vi "Read.vi"(8 "error in (no error)":errorcluster, 9 "Starting independent variables":dbl[](array[numeric]), 10 "Current independent variables":dbl[](array[numeric]), 11 "Photon Counter with LCD Reader in":refnum<class "Photon Counter with LCD Reader.lvclass">) -> (0 "error out":errorcluster, 2 "Data Channels":T1, 3 "Photon Counter with LCD Reader out":refnum<class "Photon Counter with LCD Reader.lvclass">)   [LabVIEW 2017, in "Photon Counter with LCD Reader.lvclass"]
doc: "Prepare for read, wait the time delay, and take data from up to 4 channels."
uses:
  Photon Counter with LCD Reader.lvclass
  Instruments/Utility Classes/Readable/Data Channels.ctl
  Instruments/Utility Classes/Readable/Data Channel.ctl
  Instruments/Utility Classes/Readable/Data Point.ctl
  Instruments/Utility Classes/Readable/Time.ctl
  Instruments/Utility Classes/Readable/X.ctl
  Photon Counter with LCD Reader.lvclass/Photon Counter with LCD Reader.ctl
  Reader/Reader.lvclass
  Instruments/LCD/LCD Retarder.lvclass
  Instruments/Utility Classes/Readable/Readable.lvclass
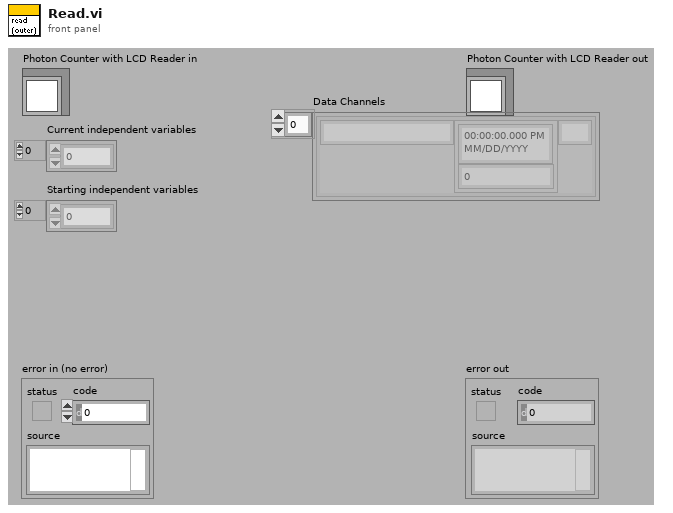
[diagram p1: front panel]
types:
  T1 = typedef "Readable.lvclass/Data Channels.ctl" = T2[]
  T2 = typedef "Readable.lvclass/Data Channel.ctl" = cluster{"Name":string, "Data Point":T3, "Unit":string}
  T3 = typedef "Readable.lvclass/Data Point.ctl" = cluster{"t":T4, "x":T5}
  T4 = typedef "Readable.lvclass/Time.ctl" = timestamp
  T5 = typedef "Readable.lvclass/X.ctl" = dbl
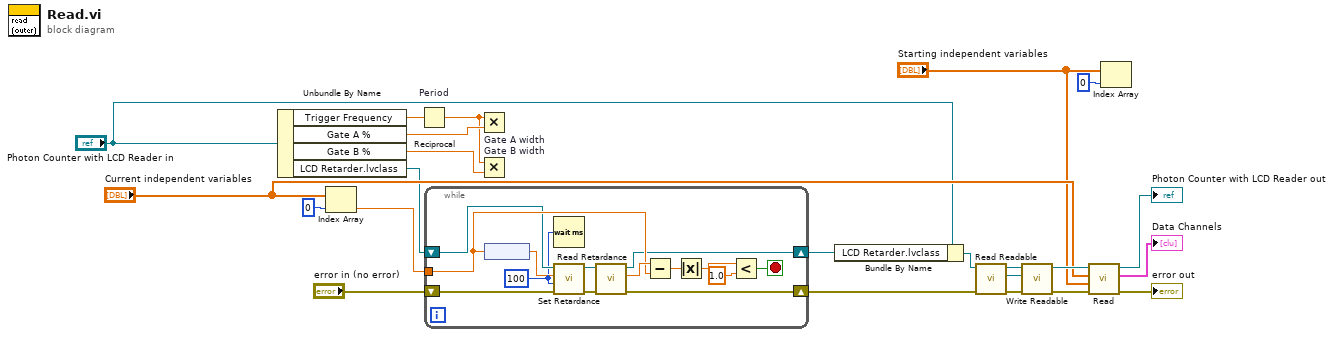
[diagram p0: block diagram]
diagram:
  n1 = Unbundle By Name("Photon Counter with LCD Reader in") -> ("Trigger Frequency"=w19:dbl[unit], "Gate A %"=w18:dbl, "Gate B %"=w17:dbl, "LCD Retarder.lvclass"=w7:refnum<class "LCD Retarder.lvclass">)
  n2 = Index Array(array="Current independent variables", index=0) -> (element=w4:dbl)
  n3 = Reciprocal "Period"(x=w19) -> (1/x=w16:dbl[unit])
  n4 = while {
    tunnel: w4 -> [w32]
    shift-right: [w29] -> w5
    shift-left: "error in (no error)" -> [w28]
    shift-right: [w30] -> w2
    shift-left: w7 -> [w26]
    stop <- w33 stop-if-true
    w24 = u32 100 ("milliseconds to wait")
    n5 = node(w32) -> (w31:dbl[unit])
    n6 = Wait (ms)(milliseconds to wait=w24) -> ()  [unwired: 1 out]
    n7 = call "Set Retardance.vi"("errorIN"=w28, "milliseconds to wait (0)"=w24, "Retardance"=w31, "LCD in"=w26) -> ("errorOUT"=w27:errorcluster, "LCD out"=w25:refnum<class "LCD Retarder.lvclass">)  [unwired: 5 in, 1 out]
    n8 = call "Read Retardance.vi"("errorIN"=w27, "LCD in"=w25) -> ("errorOUT"=w29:errorcluster, "Retardance out"=w37:dbl, "LCD out"=w30:refnum<class "LCD Retarder.lvclass">)  [unwired: 7 in]
    n9 = Subtract(x=w37, y=w32) -> (x-y=w36:dbl)
    n10 = Absolute Value(x=w36) -> (abs(x)=w35:dbl)
    n11 = Less?(x=w35, y=1.0) -> (x < y?=w33:bool)
  }
  n12 = Multiply "Gate A width"(x=w16, y=w18) -> ()  [unwired: 1 out]
  n13 = Multiply "Gate B width"(x=w16, y=w17) -> ()  [unwired: 1 out]
  n14 = Bundle By Name(cluster="Photon Counter with LCD Reader in", "LCD Retarder.lvclass"=w2) -> (w1:refnum<class "Photon Counter with LCD Reader.lvclass">)
  n15 = call-dynamic "Read Readable.vi"("error in (no error)"=w5, "Reader.lvclass in"=w1) -> ("error out"=w13:errorcluster, "Readable.lvclass"=w14:refnum<class "Readable.lvclass">, "Reader.lvclass out"=w15:refnum<class "Photon Counter with LCD Reader.lvclass">)  [unwired: 7 out]
  n16 = call-dynamic "Write Readable.vi"("error in (no error)"=w13, "Readable.lvclass"=w14, "Reader.lvclass in"=w15) -> ("error out"=w9:errorcluster, "Reader.lvclass out"=w12:refnum<class "Photon Counter with LCD Reader.lvclass">)  [unwired: 7 out]
  n17 = call-parent "Read.vi"("error in (no error)"=w9, "Starting independent variables"="Starting independent variables", "Current independent variables"="Current independent variables", "Reader in"=w12) -> ("error out"=→"error out":errorcluster, "Data Channels"=→"Data Channels":T1, "Reader out"=→"Photon Counter with LCD Reader out":refnum<class "Photon Counter with LCD Reader.lvclass">)  [unwired: 5 in]
  n18 = Index Array(array="Starting independent variables", index=0) -> ()  [unwired: 1 out]
